vi "Tabs - Page Visibility.vi"(5 "Matching Tab#":i32[](array[numeric])=[0, 1, 2, 3, 11, 12, -1, -1], 7 "PageLabel":string[](array[string])=["Setup", "Execute", "Report", "Master Data", "Admin", "Config", "Logon", "Debug"], 8 "Error In":errorcluster, 10 "[TabUserAccess]":bool[](array[boolean]), 11 "TabControl in":refnum<vi>) -> (0 "Error Out":errorcluster)   [LabVIEW 2013]
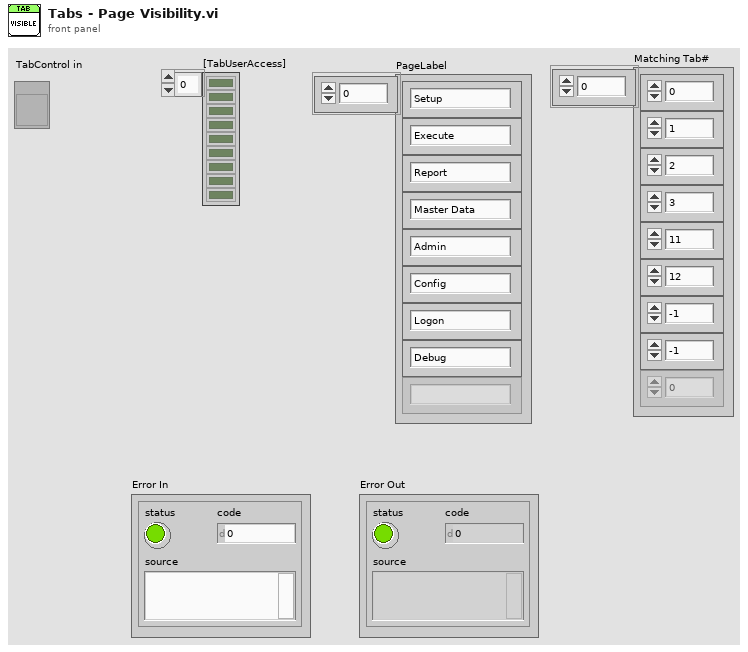
[diagram p1: front panel]
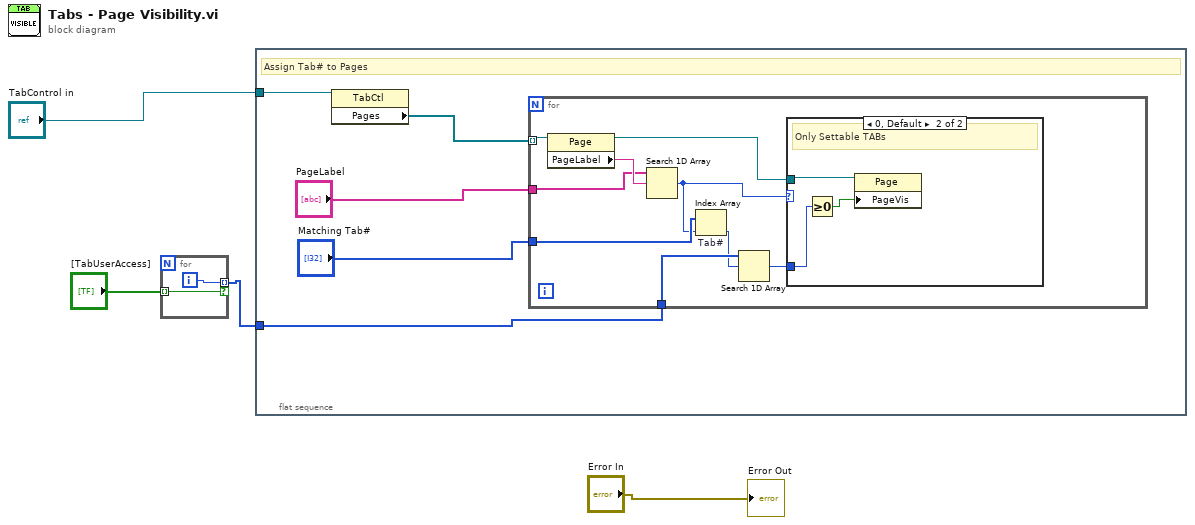
[diagram p0: block diagram]
diagram:
  n1 = for {
    tunnel: "[TabUserAccess]" -> [w5] mode=indexing
    tunnel: [w6] -> w3 mode=indexing if=w5
    i -> [w6]
  }
  n2 = flat-sequence {
    tunnel: w3 -> [w8]
    tunnel: "TabControl in" -> [w7]
    frame #0 {
      # "Assign Tab# to Pages"
      n3 = property on="Property Node" class="TabCtl"(reference=w7) -> ("Pages"=w10:refnum<vi>[])  [unwired: 1 in, 2 out]
      n4 = for {
        tunnel: w10 -> [w20] mode=indexing
        tunnel: "PageLabel" -> [w18]
        tunnel: "Matching Tab#" -> [w17]
        tunnel: w8 -> [w16]
        n5 = property class="Page"(reference=w20) -> (reference out=w15:refnum<vi>, "PageLabel"=w19:string)  [unwired: 1 in, 1 out]
        n6 = Search 1D Array(1D array=w18, element=w19) -> (index of element=w12:i32)  [unwired: 1 in]
        n7 = Index Array "Tab#"(array=w17, index=w12) -> (element=w14:i32)
        n8 = Search 1D Array(1D array=w16, element=w14) -> (index of element=w13:i32)  [unwired: 1 in]
        n9 = case shown="0, Default" w12 {
          tunnel: w15 -> [_ w22]
          tunnel: w13 -> [_ w21]
          frame -1 {
            # "Logon and Debug Set in Application"
          }
          frame 0, Default {
            # "Only Settable TABs"
            n10 = Greater Or Equal To 0?(x=w21) -> (x >= 0?=w23:bool)
            n11 = property class="Page"(reference=w22, "PageVis"=w23) -> ()  [unwired: 1 in, 2 out]
          }
        }
      }
    }
  }
  "Error Out" <- "Error In"
